vi "Set Sender.vi"(10 "Sender":refnum<class "Sender.lvclass">, 11 "Last Ack Msg in":refnum<class "Last Ack Msg.lvclass">) -> (3 "Last Ack Msg out":refnum<class "Last Ack Msg.lvclass">)   [LabVIEW 2021, in "jettl.lvlib" / "Last Ack Msg.lvlib" / "Last Ack Msg.lvclass"]
uses:
  Last Ack Msg.lvclass
  Sender/Sender/Sender.lvclass
  Last Ack Msg.lvclass/Last Ack Msg.ctl
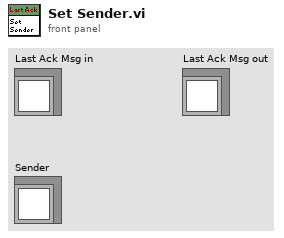
[diagram p1: front panel]
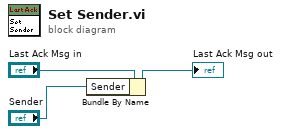
[diagram p0: block diagram]
diagram:
  n1 = Bundle By Name(cluster="Last Ack Msg in", "Sender"="Sender") -> (→"Last Ack Msg out":refnum<class "Last Ack Msg.lvclass">)
